vi "OOQMH.vi"(10 "Sharing Queue":refnum<queue>, 11 "OOQMH in":refnum<class "OOQMH.lvclass">) -> ()   [LabVIEW 2024, in "OOQMH.lvlib" / "OOQMH.lvclass"]
uses:
  OOQMH.lvclass
  Message/Message.lvclass
  OOQMH.lvclass/OOQMH.ctl
panel:
  out "error out":errorcluster
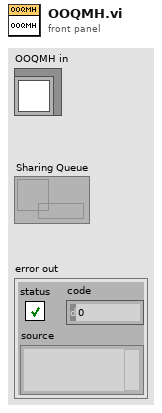
[diagram p1: front panel]
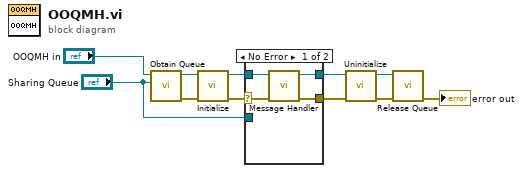
[diagram p0: block diagram]
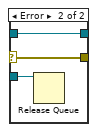
[diagram p2: hidden frame]
diagram:
  n1 = call-dynamic "Obtain Queue.vi"("Sharing Queue"="Sharing Queue", "OOQMH in"="OOQMH in") -> ("error out"=w9:errorcluster, "OOQMH out"=w10:refnum<class "OOQMH.lvclass">)  [unwired: 8 in]
  n2 = call-dynamic "Initialize.vi"("error in (no error)"=w9, "OOQMH in"=w10) -> ("error out"=w2:errorcluster, "OOQMH out"=w5:refnum<class "OOQMH.lvclass">)  [unwired: 8 in]
  n3 = case shown="No Error" w2 {
    selector: w2 -> [w12 w18]
    tunnel: w5 -> [w15 w17]
    tunnel: [w14 w18] -> w4
    tunnel: [w13 w17] -> w3
    tunnel: "Sharing Queue" -> [_ w16]
    frame No Error {
      n4 = call-dynamic "Message Handler.vi"("error in (no error)"=w12, "OOQMH in"=w15) -> ("error out"=w14:errorcluster, "OOQMH out"=w13:refnum<class "OOQMH.lvclass">)  [unwired: 8 in]
    }
    frame Error {
      n5 = Release Queue(queue=w16) -> ()  [unwired: 2 in, 3 out]
    }
  }
  n6 = call-dynamic "Uninitialize.vi"("error in (no error)"=w4, "OOQMH in"=w3) -> ("error out"=w8:errorcluster, "OOQMH out"=w7:refnum<class "OOQMH.lvclass">)  [unwired: 8 in]
  n7 = call-dynamic "Release Queue.vi"("error in (no error)"=w8, "OOQMH in"=w7) -> ("error out"=→"error out":errorcluster)  [unwired: 8 in, 1 out]
